vi "Pre Launch Init.vi"(11 "Controller In":refnum<class "Controller.lvclass">) -> (0 "Error Out":errorcluster, 3 "Controller Out":refnum<class "Controller.lvclass">)   [LabVIEW 2023, in "MVC Actors.lvlib" / "Controller.lvclass"]
doc: "(<B>Filename</B>: Actor Framework.lvlib:Actor.lvclass:Pre Launch Init.vi)\n\nDefines behavior that occurs after the Launch Nested Actor method is invoked but before the actor's Actor Core method begins running.\n\nBy default, this method does nothing. A descendant class may override it to define behavior."
uses:
  Controller.lvclass
  View Settings.ctl
  Controller.lvclass/Controller.ctl
  <vilib>/LS Instruments AG/Async Methods Actor/Async Methods Actor/Async Methods Actor/Async Methods Actor.lvclass
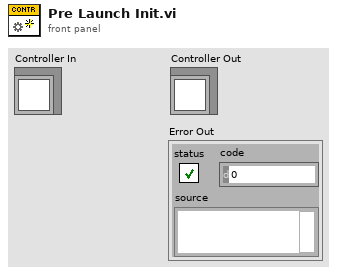
[diagram p1: front panel]
types:
  T1 = typedef "MVC Actors.lvlib/Controller.lvclass/View Settings.ctl" = cluster{"Exclude From Broadcast":bool, "Receive Only":bool, "Paused":bool}
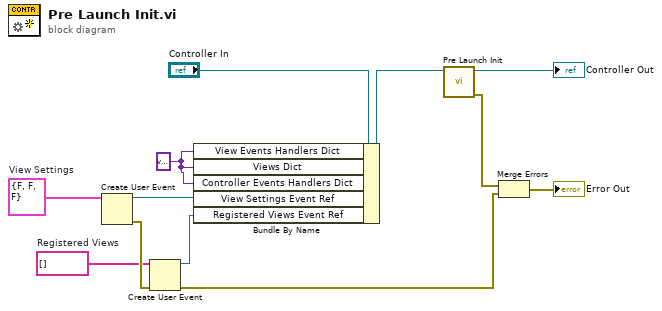
[diagram p0: block diagram]
diagram:
  w2 = string[] []  # Registered Views
  w8 = T1 {"Exclude From Broadcast"=FALSE, "Receive Only"=FALSE, "Paused"=FALSE}  # View Settings
  w1 = variant ("Events Dict")
  n1 = Create User Event(user event datatype=w8) -> (user event=w7:refnum<user-event>, error out=w3:errorcluster)  [unwired: 1 in]
  n2 = Create User Event(user event datatype=w2, error in=w3) -> (user event=w5:refnum<user-event>, error out=w4:errorcluster)
  n3 = Bundle By Name(cluster="Controller In", "View Events Handlers Dict"=w1, "Views Dict"=w1, "Controller Events Handlers Dict"=w1, "View Settings Event Ref"=w7, "Registered Views Event Ref"=w5) -> (w9:refnum<class "Controller.lvclass">)
  n4 = call-parent "Pre Launch Init.vi"("Async Methods Actor in"=w9) -> ("error out"=w10:errorcluster, "Async Methods Actor out"=→"Controller Out":refnum<class "Controller.lvclass">)  [unwired: 9 in]
  n5 = Merge Errors(w10, w4) -> (→"Error Out":errorcluster)
